vi "Create Resources.vi"() -> (4 "address space collection":refnum<class "Address Space Collection.lvclass">, 15 "acq dsp session":refnum<class "niUSRP Rx DSP v2 FPGA.lvclass">)   [LabVIEW 2025, in "niUSRP Rx DSP v2 FPGA.lvclass"]
uses:
  niUSRP Rx DSP v2 FPGA.lvclass
  C:/Program Files/NI/LVAddons/niidl/1/instr.lib/_niInstr/Instruction Framework/v1/FPGA/Interfaces/Address Space/Address Space.lvclass
  <instrlib>/_niInstr/Instruction Framework/v1/FPGA/Interfaces/Address Space Collection/Address Space Collection.lvclass
  niUSRP Rx DSP v2 FPGA.lvclass/niUSRP Rx DSP v2 FPGA.ctl
  <vilib>/rvi/DataTransferAndStorage/Container/Common/niFpgaContainerExecOnDevCompGetState.vi
  <vilib>/rvi/Emulation/niFpgaEmulationIsFPGAContextNoSignature.vi
  <vilib>/rvi/DataTransferAndStorage/Container/Common/niFpgaContainerGetUniqueNameForEmu.vi
  <vilib>/rvi/Memory/Memory_Emulation/niFpgaMemoryEmulationCacheClearOnFirstRun.vi
  <vilib>/rvi/Memory/Memory_Emulation/nirvimemoryEmulationManagerCache_MakeExclusive.vi
  <vilib>/rvi/Memory/Memory_Emulation/niFpgaMemoryEmulationValidateCache.vi
  <vilib>/rvi/Memory/Memory_Emulation/nirvimemoryEmulationManagerCache_InsertValue.vi
  <vilib>/Utility/error.llb/Clear Errors.vi
  <vilib>/rvi/Memory/Memory_Emulation/nirvimemoryEmulationManagerCache_ReleaseExclusive.vi
  <vilib>/rvi/Memory/Memory_Emulation/nirvimemoryEmulationManagerCache_GetValue.vi
  <vilib>/rvi/Memory/Memory_Emulation/nirvimemoryEmulationManagerCache_SetValue.vi
  <vilib>/rvi/Emulation/niFpgaProcessEmulError.vi
  <vilib>/rvi/Emulation/niFpgaSctlEmulationGetInTimedLoop.vi
  <vilib>/rvi/DataTransferAndStorage/Container/XNode/niFpgaContainer.xnode
  <vilib>/rvi/DataTransferAndStorage/Register/Emulation/niFpgaRegisterEmulationRefIn.vi
  <instrlib>/_niInstr/Basic Elements/v1/FPGA/niInstr Basic Elements v1 FPGA.lvlib
  <instrlib>/_niInstr/Instruction Framework/v1/FPGA/Collection Builder/Collection Builder.lvclass
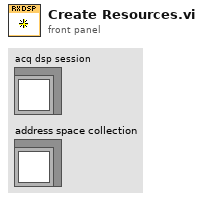
[diagram p1: front panel]
types:
  T1 = typedef "niInstr Address Space Collection Builder v1 FPGA.lvlib/Parent Metadata.ctl" = cluster{"UID":u16, "version":u16, "oldest compatible version":u16}
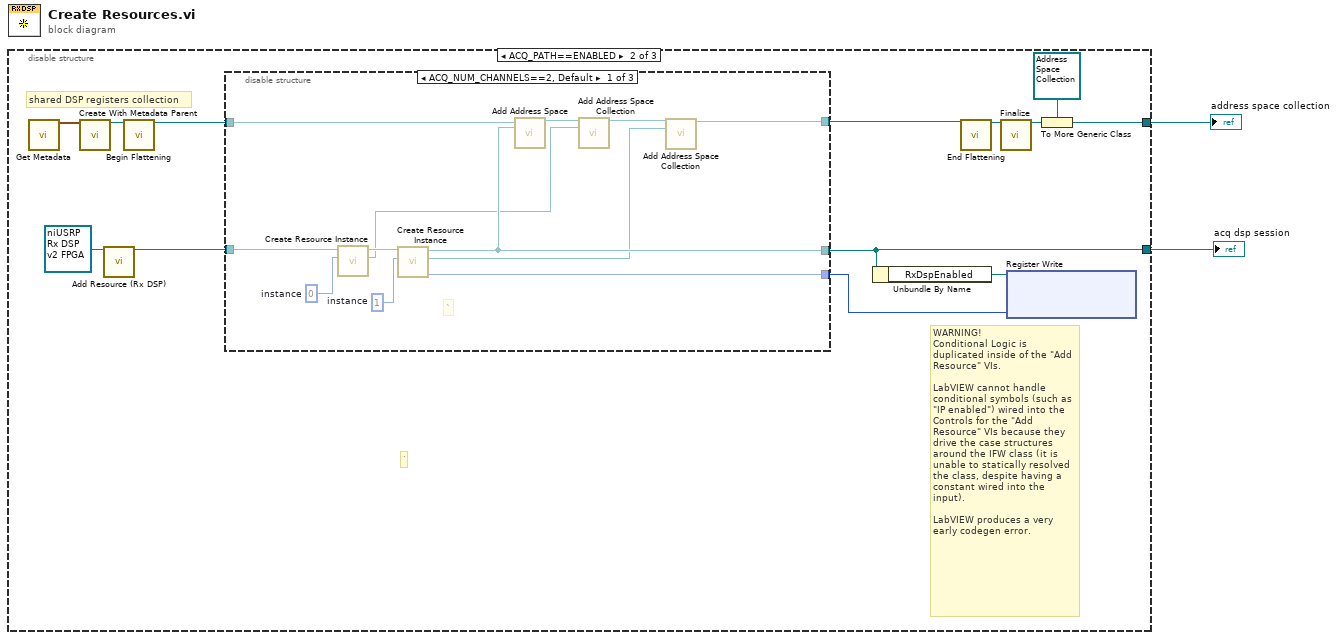
[diagram p0: block diagram]
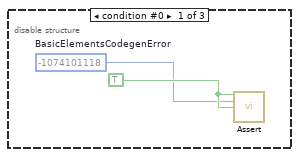
[diagram p2: hidden frame]
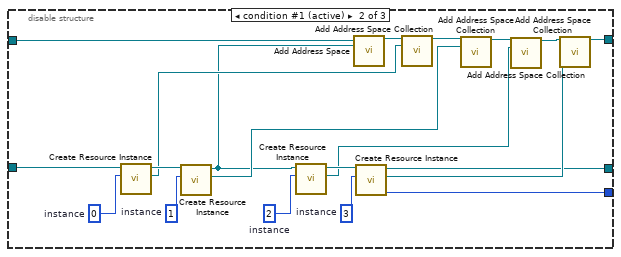
[diagram p3: hidden frame]
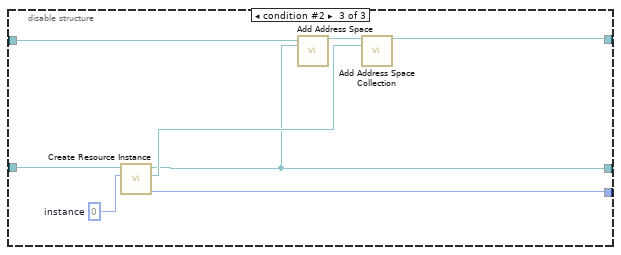
[diagram p4: hidden frame]
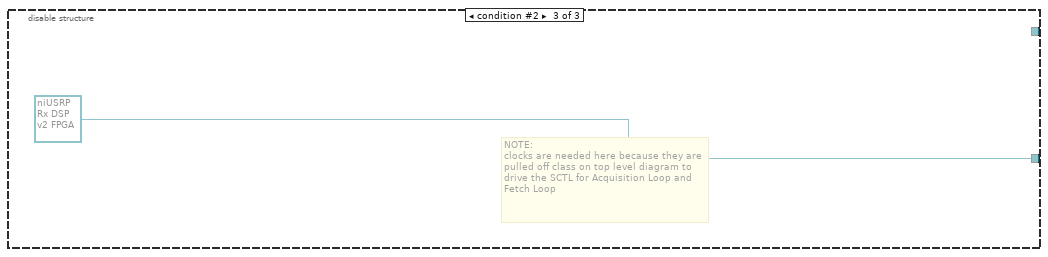
[diagram p5: hidden frame]
diagram:
  n1 = disable-structure shown="ACQ_PATH==ENABLED" {
    disable-tunnel: [_ w7 refnum<class "niUSRP Rx DSP v2 FPGA.lvclass"> refnum ("acq")] -> w2
    disable-tunnel: [_ w14 _] -> w1
    frame condition #0 {
      w4 = TRUE ("assert")
      w3 = -1074101118  # BasicElementsCodegenError
      n2 = call <instrlib>:"Assert.vi"("assert"=w4, "error code"=w3, "enable show error"=w4) -> ()  [unwired: 13 in]
    }
    frame condition #1 (active) {
      # "`"
      # "shared DSP registers collection"
      # "WARNING!\nConditional Logic is duplicated inside of the \"Add Resource\" VIs.\n\nLabVIEW cannot handle conditional symbols (such as \"IP enabled\") wired into the Controls for the \"Add Resource\" VIs because they drive the case structures around the IFW class (it is unable to statically resolved the class, despite having a constant wired into the input).\n\nLabVIEW produces a very early codegen error."
      n3 = call "Get Metadata.vi"() -> ("acq metadata"=w17:T1)  [unwired: 15 in]
      n4 = call <instrlib>:"Create With Metadata Parent.vi"("parent metadata"=w17) -> ("collection builder"=w16:refnum<class "Collection Builder.lvclass">)  [unwired: 14 in]
      n5 = call "Add Resource (Rx DSP).vi"("acq in"=refnum<class "niUSRP Rx DSP v2 FPGA.lvclass"> refnum ("acq")) -> ("output cluster"=w10:refnum<class "niUSRP Rx DSP v2 FPGA.lvclass">)  [unwired: 14 in]
      n6 = call <instrlib>:"Begin Flattening.vi"("collection builder in"=w16) -> ("collection builder out"=w9:refnum<class "Collection Builder.lvclass">)  [unwired: 14 in]
      n7 = disable-structure shown="ACQ_NUM_CHANNELS==2, Default" {
        disable-tunnel: w10 -> [w29 w49 w57]
        disable-tunnel: [w26 w31 w52] -> w7
        disable-tunnel: w9 -> [w19 w41 w53]
        disable-tunnel: [w20 w35 w51] -> w8
        disable-tunnel: [w18 w30 w50] -> w5
        frame condition #0 {
          w25 = u8 1  # instance
          w28 = u8 0  # instance
          # "`"
          n8 = call "Create Resource Instance.vi"("instance"=w28, "niUSRP Rx DSP v2 FPGA in"=w29) -> ("address space collection"=w21:refnum<class "Address Space Collection.lvclass">, "niUSRP Rx DSP v2 FPGA out"=w27:refnum<class "niUSRP Rx DSP v2 FPGA.lvclass">)  [unwired: 7 in, 1 out]
          n9 = call "Create Resource Instance.vi"("instance"=w25, "niUSRP Rx DSP v2 FPGA in"=w27) -> ("RxDspSupport"=w18:u64, "address space collection"=w22:refnum<class "Address Space Collection.lvclass">, "niUSRP Rx DSP v2 FPGA out"=w26:refnum<class "niUSRP Rx DSP v2 FPGA.lvclass">)  [unwired: 7 in]
          n10 = call <instrlib>:"Add Address Space.vi"("collection builder in"=w19, "address space"=w26) -> ("collection builder out"=w23:refnum<class "Collection Builder.lvclass">)  [unwired: 13 in]
          n11 = call <instrlib>:"Add Address Space Collection.vi"("collection builder in"=w23, "address space collection"=w21) -> ("collection builder out"=w24:refnum<class "Collection Builder.lvclass">)  [unwired: 13 in]
          n12 = call <instrlib>:"Add Address Space Collection.vi"("collection builder in"=w24, "address space collection"=w22) -> ("collection builder out"=w20:refnum<class "Collection Builder.lvclass">)  [unwired: 13 in]
        }
        frame condition #1 (active) {
          w40 = u8 3  # instance
          w38 = u8 2  # instance
          w46 = u8 1  # instance
          w48 = u8 0  # instance
          n13 = call "Create Resource Instance.vi"("instance"=w48, "niUSRP Rx DSP v2 FPGA in"=w49) -> ("address space collection"=w42:refnum<class "Address Space Collection.lvclass">, "niUSRP Rx DSP v2 FPGA out"=w47:refnum<class "niUSRP Rx DSP v2 FPGA.lvclass">)  [unwired: 7 in, 1 out]
          n14 = call "Create Resource Instance.vi"("instance"=w46, "niUSRP Rx DSP v2 FPGA in"=w47) -> ("address space collection"=w43:refnum<class "Address Space Collection.lvclass">, "niUSRP Rx DSP v2 FPGA out"=w32:refnum<class "niUSRP Rx DSP v2 FPGA.lvclass">)  [unwired: 7 in, 1 out]
          n15 = call "Create Resource Instance.vi"("instance"=w38, "niUSRP Rx DSP v2 FPGA in"=w32) -> ("address space collection"=w34:refnum<class "Address Space Collection.lvclass">, "niUSRP Rx DSP v2 FPGA out"=w39:refnum<class "niUSRP Rx DSP v2 FPGA.lvclass">)  [unwired: 7 in, 1 out]
          n16 = call <instrlib>:"Add Address Space.vi"("collection builder in"=w41, "address space"=w32) -> ("collection builder out"=w44:refnum<class "Collection Builder.lvclass">)  [unwired: 13 in]
          n17 = call "Create Resource Instance.vi"("instance"=w40, "niUSRP Rx DSP v2 FPGA in"=w39) -> ("RxDspSupport"=w30:u64, "address space collection"=w33:refnum<class "Address Space Collection.lvclass">, "niUSRP Rx DSP v2 FPGA out"=w31:refnum<class "niUSRP Rx DSP v2 FPGA.lvclass">)  [unwired: 7 in]
          n18 = call <instrlib>:"Add Address Space Collection.vi"("collection builder in"=w44, "address space collection"=w42) -> ("collection builder out"=w45:refnum<class "Collection Builder.lvclass">)  [unwired: 13 in]
          n19 = call <instrlib>:"Add Address Space Collection.vi"("collection builder in"=w45, "address space collection"=w43) -> ("collection builder out"=w37:refnum<class "Collection Builder.lvclass">)  [unwired: 13 in]
          n20 = call <instrlib>:"Add Address Space Collection.vi"("collection builder in"=w37, "address space collection"=w34) -> ("collection builder out"=w36:refnum<class "Collection Builder.lvclass">)  [unwired: 13 in]
          n21 = call <instrlib>:"Add Address Space Collection.vi"("collection builder in"=w36, "address space collection"=w33) -> ("collection builder out"=w35:refnum<class "Collection Builder.lvclass">)  [unwired: 13 in]
        }
        frame condition #2 {
          w56 = u8 0  # instance
          n22 = call "Create Resource Instance.vi"("instance"=w56, "niUSRP Rx DSP v2 FPGA in"=w57) -> ("RxDspSupport"=w50:u64, "address space collection"=w54:refnum<class "Address Space Collection.lvclass">, "niUSRP Rx DSP v2 FPGA out"=w52:refnum<class "niUSRP Rx DSP v2 FPGA.lvclass">)  [unwired: 7 in]
          n23 = call <instrlib>:"Add Address Space.vi"("collection builder in"=w53, "address space"=w52) -> ("collection builder out"=w55:refnum<class "Collection Builder.lvclass">)  [unwired: 13 in]
          n24 = call <instrlib>:"Add Address Space Collection.vi"("collection builder in"=w55, "address space collection"=w54) -> ("collection builder out"=w51:refnum<class "Collection Builder.lvclass">)  [unwired: 13 in]
        }
      }
      n25 = Unbundle By Name(w7) -> ("RxDspEnabled"=w6:refnum<k21>)
      n26 = call <instrlib>:"End Flattening.vi"("collection builder in"=w8) -> ("collection builder out"=w12:refnum<class "Collection Builder.lvclass">)  [unwired: 14 in]
      n27 = call <instrlib>:"Finalize.vi"("collection builder in"=w12) -> ("address space collection"=w11:refnum<class "Address Space Collection.lvclass">)  [unwired: 14 in]
      n28 = xnode ("Register Write")("Data"=w5, "Register In"=w6) -> ()  [unwired: 1 out]
      n29 = To More Generic Class(target class=refnum<class "Address Space Collection.lvclass"> refnum ("collection"), reference=w11) -> (generic class reference=w14:refnum<class "Address Space Collection.lvclass">)
    }
    frame condition #2 {
      # "NOTE:\nclocks are needed here because they are pulled off class on top level diagram to drive the SCTL for Acquisition Loop and Fetch Loop"
    }
  }
  "acq dsp session" <- w2
  "address space collection" <- w1
